vi "dfd_Build CIC Parameters.vi"(8 "fpass":dbl, 9 "stop band attenuation [dB]":dbl, 11 "CIC factor":i32) -> (3 "CIC stage":i32)   [LabVIEW 2017, in "NI_DigFilterLicensed.lvlib"]
uses:
  <vilib>/addons/Digital Filter Design/NI_DigFilterLicensed.lvlib
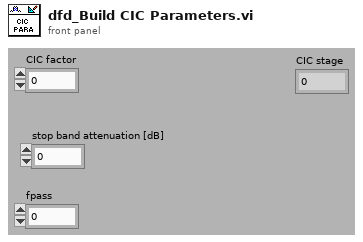
[diagram p1: front panel]
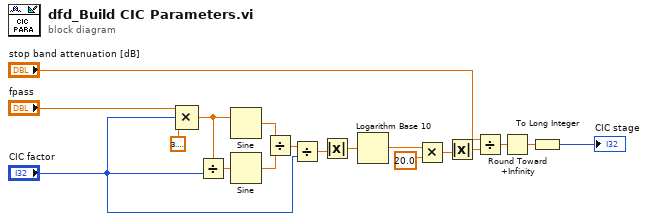
[diagram p0: block diagram]
diagram:
  n1 = Compound Arithmetic op=MULTIPLY("fpass", "CIC factor", 3.141592653589793) -> (w17:dbl)
  n2 = Divide(x=w17, y="CIC factor") -> (x/y=w13:dbl)
  n3 = Sine(x=w17) -> (sin(x)=w14:dbl)
  n4 = Sine(x=w13) -> (sin(x)=w15:dbl)
  n5 = Divide(x=w14, y=w15) -> (x/y=w16:dbl)
  n6 = Divide(x=w16, y="CIC factor") -> (x/y=w9:dbl)
  n7 = Absolute Value(x=w9) -> (abs(x)=w6:dbl)
  n8 = Logarithm Base 10(1:w6) -> (0:w4:dbl)
  n9 = Multiply(x=w4, y=20.0) -> (x*y=w5:dbl)
  n10 = Absolute Value(x=w5) -> (abs(x)=w1:dbl)
  n11 = Divide(x="stop band attenuation [dB]", y=w1) -> (x/y=w12:dbl)
  n12 = Round Toward +Infinity(x=w12) -> (ceil(x): smallest int >= x=w11:dbl)
  n13 = To Long Integer(number=w11) -> (32bit integer=→"CIC stage":i32)
